vi "sem_open.vi"(7 "permissions (0664)":T1={"owner"={"read"=TRUE, "write"=TRUE, "execute"=FALSE}, "group"={"read"=TRUE, "write"=TRUE, "execute"=FALSE}, "everyone"={"read"=TRUE, "write"=FALSE, "execute"=FALSE}}, 8 "error in (no error)":errorcluster, 9 "initial value (0)":u32, 10 "flags":T2[](array[typedef]) items=["O_RDONLY"=0, "O_WRONLY"=1, "O_RDWR"=2, "O_CREAT"=64, "O_EXCL"=128, "O_TRUNC"=512], 11 "name":string) -> (0 "error out":errorcluster, 3 "semaphore ptr out":u64)   [LabVIEW 2016, in "Linux RT IPC.POSIX Threads.lvlib" / "POSIX Thread Object.lvclass"]
uses:
  POSIX Thread Object.lvclass
  C/Controls/file creation flags.ctl
  Controls/pthread functions.ctl
  <vilib>/NI/NI Linux RT Errno/Linux Errno.lvlib
  C/Linux RT IPC.C.lvlib
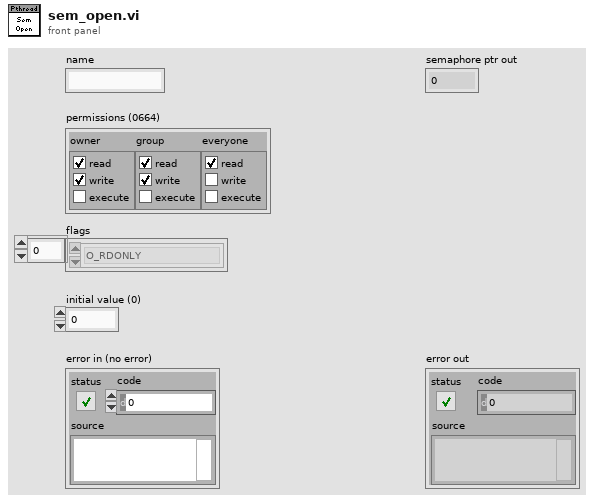
[diagram p1: front panel]
types:
  T1 = cluster{"owner":cluster{"read":bool, "write":bool, "execute":bool}, "group":cluster{"read":bool, "write":bool, "execute":bool}, "everyone":cluster{"read":bool, "write":bool, "execute":bool}}
  T2 = typedef "Linux RT IPC.C.lvlib/file creation flags.ctl" = u32
  T3 = typedef "Linux RT IPC.POSIX Threads.lvlib/POSIX Thread Object.lvclass/pthread functions.ctl" = enum16{"unspecified", "pthread_condattr_init", "pthread_condattr_destroy", "pthread_condattr_getclock", "pthread_condattr_setclock", "pthread_condattr_getpshared", "pthread_condattr_setpshared", "pthread_cond_init", "pthread_cond_destroy", "pthread_cond_broadcast", "pthread_cond_signal", "pthread_cond_timedwait", "pthread_cond_wait", "pthread_mutexattr_init", "pthread_mutexattr_destroy", "pthread_mutexattr_getprioceiling", "pthread_mutexattr_setprioceiling", "pthread_mutexattr_getprotocol", "pthread_mutexattr_setprotocol", "pthread_mutexattr_getpshared", "pthread_mutexattr_setpshared", "pthread_mutexattr_gettype", "pthread_mutexattr_settype", "pthread_mutex_init", "pthread_mutex_destroy", "pthread_mutex_getprioceiling", "pthread_mutex_setprioceiling", "pthread_mutex_lock", "pthread_mutex_timedlock", "pthread_mutex_trylock", "pthread_mutex_unlock", "sem_destroy", "sem_getvalue", "sem_init", "sem_open", "sem_post", "sem_timedwait", "sem_trywait", "sem_wait", "barrier_init", "barrier_destroy", "barrier_wait", "barrierattr_init", "barrierattr_destroy", "barrierattr_getpshared", "barrierattr_setpshared"}
  T4 = typedef "Linux Errno.lvlib/errno.ctl" = enum16{"NO ERROR", "EPERM", "ENOENT", "ESRCH", "EINTR", "EIO", "ENXIO", "E2BIG", "ENOEXEC", "EBADF", "ECHILD", "EAGAIN", "ENOMEM", "EACCES", "EFAULT", "ENOTBLK", "EBUSY", "EEXIST", "EXDEV", "ENODEV", "ENOTDIR", "EISDIR", "EINVAL", "ENFILE", "EMFILE", "ENOTTY", "ETXTBSY", "EFBIG", "ENOSPC", "ESPIPE", "EROFS", "EMLINK", "EPIPE", "EDOM", "ERANGE", "EDADLK", "ENAMETOOLONG", "ENOLCK", "ENOSYS", "ENOTEMPTY", "ELOOP", "EWOULDBLOCK", "ENOMSG", "EIDRM", "ECHRNG", "EL2NSYNC", "EL3HLT", "EL3RST", "ELNRNG", "EUNATCH", "ENOCSI", "EL2HLT", "EBADE", "EBADR", "EXFULL", "ENOANO", "EBADRQC", "EBADSLT", "EDEADLOCK", "EBFONT", "ENOSTR", "ENODATA", "ETIME", "ENOSR", "ENONET", "ENOPKG", "EREMOTE", "ENOLINK", "EADV", "ESRMNT", "ECOMM", "EPROTO", "EMULTIHOP", "EDOTDOT", "EBADMSG", "EOVERFLOW", "ENOTUNIQ", "EBADFD", "EREMCHG", "ELIBACC", "ELIBBAD", "ELIBSCN", "ELIBMAX", "ELIBEXEC", "ELISEQ", "ERESTART", "ESTRPIPE", "EUSERS", "ENOTSOCK", "EDESTADDRREQ", "EMSGSIZE", "EPROTOTYPE", "ENOPROTOOPT", "EPROTONOSUPPORT", "ESOCKTNOSUPPORT", "EOPNOTSUPP", "EPFNOSUPPORT", "EAFNOSUPPORT", "EADDRINUSE", "EADDRNOTAVAIL", "ENETDOWN", "ENETUNREACH", "ENETRESET", "ECONNABORTED", "ECONNRESET", "ENOBUFS", "EISCONN", "ENOTCONN", "ESHUTDOWN", "ETOOMANYREFS", "ETIMEDOUT", "ECONNREFUSED", "EHOSTDOWN", "EHOSTUNREACH", "EALREADY", "EINPROGRESS", "ESTALE", "EUCLEAN", "ENOTNAM", "ENAVAIL", "EISNAM", "EREMOTEIO", "EDQUOT", "ENOMEDIUM", "EMEDIUMTYPE", "ECANCELED", "ENOKEY", "EKEYEXPIRED", "EKEYREVOKED", "EKEYREJECTED", "EOWNERDEAD", "ENOTRECOVERABLE", "ERFKILL", "EHWPOISON", "UNDEFINED"}
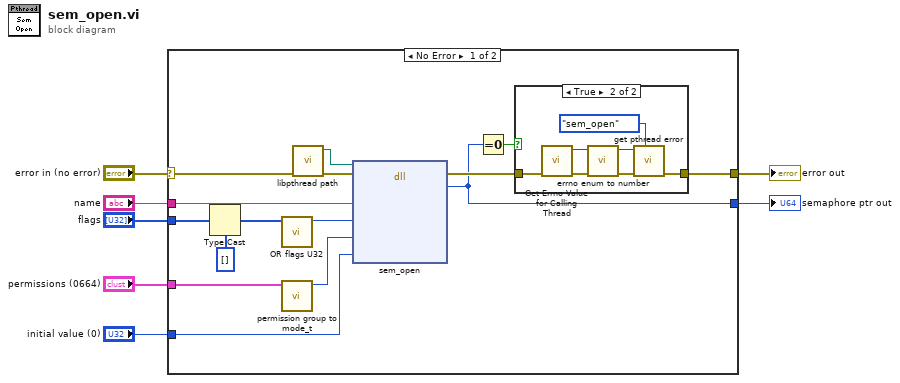
[diagram p0: block diagram]
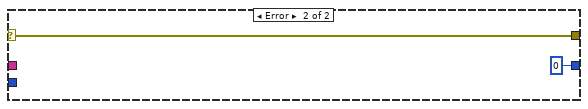
[diagram p3: hidden frame]
diagram:
  n1 = case shown="No Error" "error in (no error)" {
    selector: "error in (no error)" -> [w22 w32]
    tunnel: [w18 w32] -> w6
    tunnel: [w15 u64 0 ("pointer")] -> w5
    tunnel: "name" -> [w17 _]
    tunnel: "initial value (0)" -> [w9 _]
    tunnel: "permissions (0664)" -> [w13 _]
    tunnel: "flags" -> [w8 _]
    frame No Error {
      n2 = Type Cast(type=u32[] [], x=w8) -> (*(type *) &x=w12:u32[])
      n3 = call "OR flags U32.vi"("flags"=w12) -> ("OR'ed flags"=w10:u32)  [unwired: 10 in]
      n4 = call "permission group to mode_t.vi"("permissions group"=w13) -> ("mode_t"=w14:u32)  [unwired: 10 in]
      n5 = call "libpthread path.vi"("error in (no error)"=w22) -> ("error out"=w20:errorcluster, "path to libpthread"=w21:path)  [unwired: 9 in]
      n6 = dll-call lib="?" fn="sem_open"(path in=w21, error in=w20, "name"=w17, "oflag"=w10, "mode"=w14, "value"=w9) -> (error out=w19:errorcluster, "pointer"=w15:u64)  [unwired: 5 in, 1 out]
      n7 = Equal To 0?(x=w15) -> (x = 0?=w16:bool)
      n8 = case shown="True" w16 {
        tunnel: w19 -> [w23 w30]
        tunnel: [w23 w28] -> w18
        frame False {
        }
        frame True {
          n9 = call <vilib>:"Get Errno Value for Calling Thread.vi"("error in (no error)"=w30) -> ("error out"=w27:errorcluster, "errno"=w26:T4)  [unwired: 9 in]
          n10 = call <vilib>:"errno enum to number.vi"("error in (no error)"=w27, "errno enum"=w26) -> ("error out"=w24:errorcluster, "errno number"=w25:i32)  [unwired: 8 in]
          n11 = call "get pthread error.vi"("function"=pthread_functions."sem_open", "error in (no error)"=w24, "errno"=w25) -> ("error out"=w28:errorcluster)  [unwired: 8 in]
        }
      }
    }
    frame Error {
    }
  }
  "error out" <- w6
  "semaphore ptr out" <- w5
